vi "Disconnect.vi"(8 "error in (no error)":errorcluster, 11 "Hamamatsu_Camera in":refnum<class "Hamamatsu_Camera.lvclass">) -> (0 "error out":errorcluster, 3 "Hamamatsu_Camera out":refnum<class "Hamamatsu_Camera.lvclass">)   [LabVIEW 2023, in "CameraLibrary.lvlib" / "Hamamatsu_Camera.lvlib" / "Hamamatsu_Camera.lvclass"]
uses:
  Hamamatsu_Camera.lvclass
  Interfaces/InitDeinitInterface/InitDeinitComm Messages/Disconnected Msg/Disconnected Msg.lvclass
  <vilib>/ActorFramework/Actor/Actor.lvclass
  C:/Program Files/National Instruments/LabVIEW 2023/vi.lib/ActorFramework/Actor/Actor.lvclass
  C:/Users/quantum/Documents/LVDAQ/ConcreteClasses/ConcreteInstrumentClasses/CameraClasses/Hama_LV/HamaCam/Hamamatsu_Camera.lvclass
  C:/Users/quantum/Documents/LVDAQ/Interfaces/AbstractInstrumentClasses/Cameras_LV/CameraInterface/CameraInterface.lvclass
  C:/Users/quantum/Documents/LVDAQ/Interfaces/InitDeinitInterface/InitDeinit/InitDeinit.lvclass
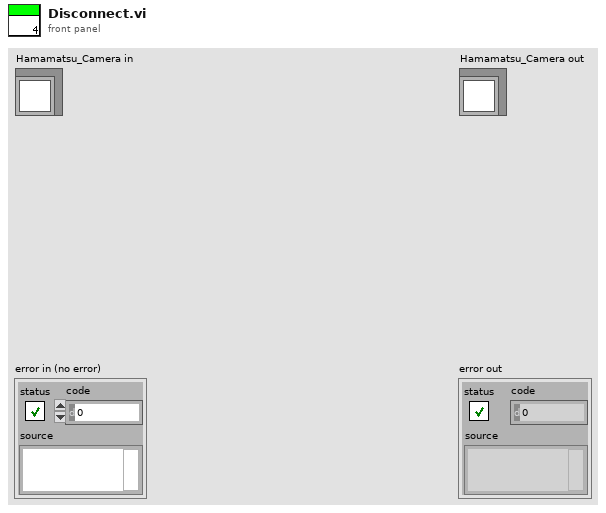
[diagram p1: front panel]
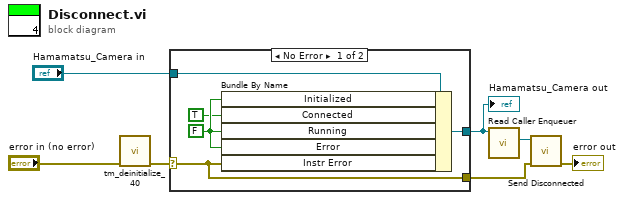
[diagram p0: block diagram]
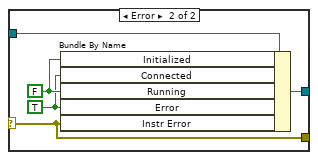
[diagram p2: hidden frame]
diagram:
  n1 = call "tm_deinitialize_40.vi"("error in (no error)"="error in (no error)") -> ("error out"=w4:errorcluster)  [unwired: 10 in]
  n2 = case shown="No Error" w4 {
    selector: w4 -> [w8 w13]
    tunnel: "Hamamatsu_Camera in" -> [w12 w17]
    tunnel: [w9 w15] -> w2
    tunnel: [w8 w13] -> w1
    frame No Error {
      w11 = FALSE ("InstrumentData.CurrentState.Initialized")
      n3 = Bundle By Name(cluster=w12, "Initialized"=w11, "Connected"=TRUE ("InstrumentData.CurrentState.Connected"), "Running"=w11, "Error"=w11, "Instr Error"=w8) -> (w9:refnum<class "Hamamatsu_Camera.lvclass">)
    }
    frame Error {
      w14 = TRUE ("InstrumentData.CurrentState.Connected")
      w16 = FALSE ("InstrumentData.CurrentState.Initialized")
      n4 = Bundle By Name(cluster=w17, "Initialized"=w16, "Connected"=w14, "Running"=w16, "Error"=w14, "Instr Error"=w13) -> (w15:refnum<class "Hamamatsu_Camera.lvclass">)
    }
  }
  "Hamamatsu_Camera out" <- w2
  n5 = call <vilib>:"Read Caller Enqueuer.vi"("Actor"=w2) -> ("Caller Enqueuer"=w7:refnum<class "Message Enqueuer.lvclass">)  [unwired: 10 in]
  n6 = call "Send Disconnected.vi"("error in (no error)"=w1, "Message Enqueuer"=w7) -> ("error out"=→"error out":errorcluster)  [unwired: 8 in, 1 out]
